vi "Template Pattern - Caller.vi"(4 "Message Size":T2 {"Message Width" min=-1 step=1; "Message Height" min=-1 step=1}, 6 "Theme":refnum<class "Theme.lvclass">, 7 "standard":T1="info", 8 "error in (no error)":errorcluster, 9 "Graphic":path, 10 "Message":string, 11 "Pop-Up in":refnum<class "Gif Parent.lvclass">) -> (0 "error out":errorcluster, 3 "Pop-Up out":refnum<class "Gif Parent.lvclass">)   [LabVIEW 2021, in "Pop-Up.lvlib" / "Gif Parent.lvclass"]
doc: "Template Pattern to be used when loading a Display Pop Up\n\n<b>Code Developed By:</b>\nDaniel Coons\nTechnology Service Corporation\n1983 S Liberty Drive\nBloomington, IN 47403\nPhone: 812 558-7100\ndaniel.coons@tsc.com\nwww.tsc.com/atcs"
uses:
  Gif Parent.lvclass
  C:/Development/TSC.Pop-Up/Popup/Popup.lvclass
  Theme/Theme.lvclass
  Popup/message info--typedef.ctl
  Graphics.ctl
  Popup/Popup.lvclass/Popup.ctl
  Popup/Data Member Access/Read Theme.vi
  Popup/Data Member Access/Write Theme.vi
  Popup/Data Member Access/Write Pic Width.vi
  Popup/Data Member Access/Write Pic Height.vi
  Popup/Data Member Access/Write Message Size.vi
  Popup/Popup.lvclass
  Pop-Up.lvlib
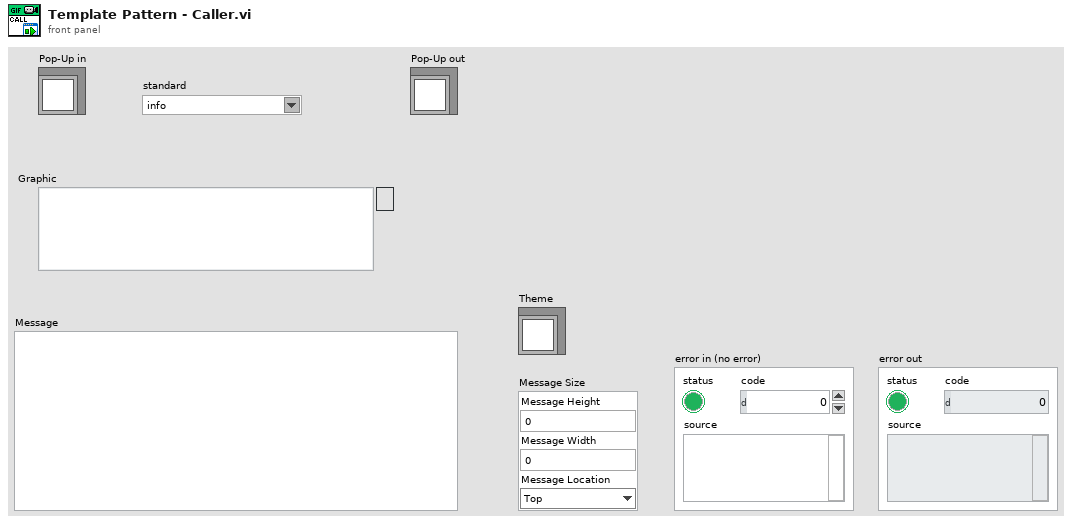
[diagram p1: front panel]
types:
  T1 = typedef "Pop-Up.lvlib/Graphics.ctl" = string
  T2 = typedef "Pop-Up.lvlib/Popup.lvclass/message info--typedef.ctl" = cluster{"Message Height":i32, "Message Width":i32, "Message Location":enum16{"Top", "Bottom", "Right", "Left"}}
  T3 = typedef "imagedata.ctl" = cluster{"image type":i32, "image depth":i32, "image":u8[], "mask":u8[], "colors":u32[], "Rectangle":cluster{"left":i16, "top":i16, "right":i16, "bottom":i16}}
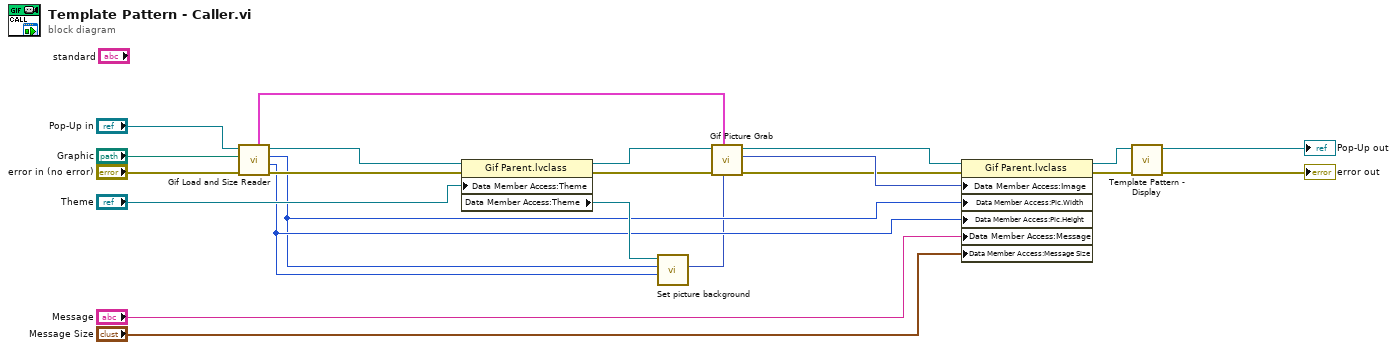
[diagram p0: block diagram]
diagram:
  n1 = call "Gif Load and Size Reader.vi"("error in (no error)"="error in (no error)", "Graphic"="Graphic", "Pop-Up.lvlib:Gif Parent.lvclass"="Pop-Up in") -> ("error out"=w14:errorcluster, "pic height"=w13:i16, "pic width"=w12:i16, "Pop-Up.lvlib:Gif Parent.lvclass out"=w18:refnum<class "Gif Parent.lvclass">, "Images"=w19:T3[])  [unwired: 4 in]
  n2 = property class="Gif Parent.lvclass"(reference=w18, error in=w14, "Data Member Access:Theme"="Theme") -> (reference out=w20:refnum<class "Gif Parent.lvclass">, error out=w15:errorcluster, "Data Member Access:Theme"=w17:refnum<class "Theme.lvclass">)
  n3 = call "Set picture background.vi"("pic height"=w13, "pic width"=w12, "Theme in"=w17) -> ("background"=w8:picture)  [unwired: 6 in, 2 out]
  n4 = call "Gif Picture Grab.vi"("picture background"=w8, "images"=w19, "error in (no error)"=w15, "Pop-Up.lvlib:Gif Parent.lvclass"=w20) -> ("error out"=w3:errorcluster, "1st picture"=w7:picture, "Pop-Up.lvlib:Gif Parent.lvclass out"=w21:refnum<class "Gif Parent.lvclass">)  [unwired: 5 in]
  n5 = property class="Gif Parent.lvclass"(reference=w21, error in=w3, "Data Member Access:Image"=w7, "Data Member Access:Pic.Width"=w12, "Data Member Access:Pic.Height"=w13, "Data Member Access:Message"="Message", "Data Member Access:Message Size"="Message Size") -> (reference out=w4:refnum<class "Gif Parent.lvclass">, error out=w1:errorcluster)
  n6 = call "Template Pattern - Display.vi"("error in (no error)"=w1, "PopUp in"=w4) -> ("error out"=→"error out":errorcluster, "PopUp out"=→"Pop-Up out":refnum<class "Gif Parent.lvclass">)  [unwired: 8 in]
